vi "TestCode.vi"() -> ()   [LabVIEW 2018]
panel:
  out "Wavelength 2":dbl caption="Wavelength"
  in  "Wavelength":dbl=930.0 caption="Wavelength (0.0)"
  out "Average Time":dbl
  in  "Average Time (0.0)":dbl=0.1
  out "Sensor Name":string
  out "Power":dbl
  out "error out":errorcluster
  in  "error in (no error)":errorcluster {"code" format="%.0x"}
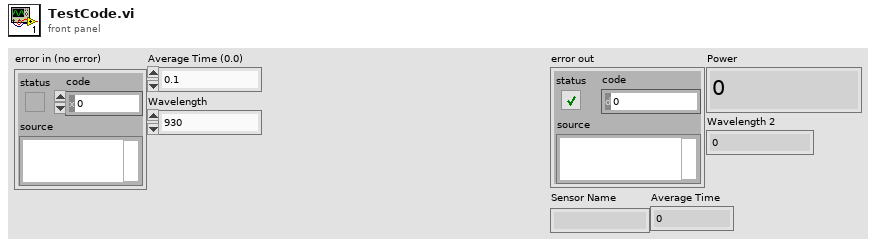
[diagram p1: front panel]
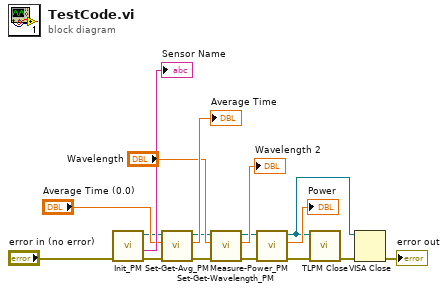
[diagram p0: block diagram]
diagram:
  n1 = call "Init_PM.vi"("error in (no error)"="error in (no error)") -> ("error out"=w16:errorcluster, "Sensor Name"=→"Sensor Name":string, "instrument handle out"=w7:refnum<visa-resource-name>)  [unwired: 8 in]
  n2 = call "Set-Get-Avg_PM.vi"("error in (no error)"=w16, "Average Time (0.0)"="Average Time (0.0)", "instrument handle"=w7) -> ("error out"=w15:errorcluster, "Average Time"=→"Average Time":dbl, "instrument handle out"=w6:refnum<visa-resource-name>)  [unwired: 6 in]
  n3 = call "Set-Get-Wavelength_PM.vi"("error in (no error)"=w15, "Wavelength"="Wavelength", "instrument handle"=w6) -> ("error out"=w14:errorcluster, "Wavelength"=→"Wavelength 2":dbl, "instrument handle out"=w5:refnum<visa-resource-name>)  [unwired: 6 in]
  n4 = call "Measure-Power_PM.vi"("error in (no error)"=w14, "instrument handle"=w5) -> ("error out"=w4:errorcluster, "Power"=→"Power":dbl, "instrument handle out"=w1:refnum<visa-resource-name>)  [unwired: 7 in]
  n5 = call "TLPM Close.vi"("error in (no error)"=w4, "instrument handle"=w1) -> ("error out"=w3:errorcluster)  [unwired: 9 in]
  n6 = VISA Close(VISA resource name=w1, error in (no error)=w3) -> (error out=→"error out":errorcluster)
